vi "SDCP SMF Receiver and Transmitter - Live Plot - Obtain Data Points.vi"(4 "error in (no error)":errorcluster, 5 "Plot file path":path, 6 "Command":enum16{"Initialize", "Acquire", "Save"}(ring), 7 "Raw frame":T1) -> (0 "error out":errorcluster)   [LabVIEW 2020]
uses:
  <vilib>/Utility/file.llb/Write Delimited Spreadsheet (string).vi
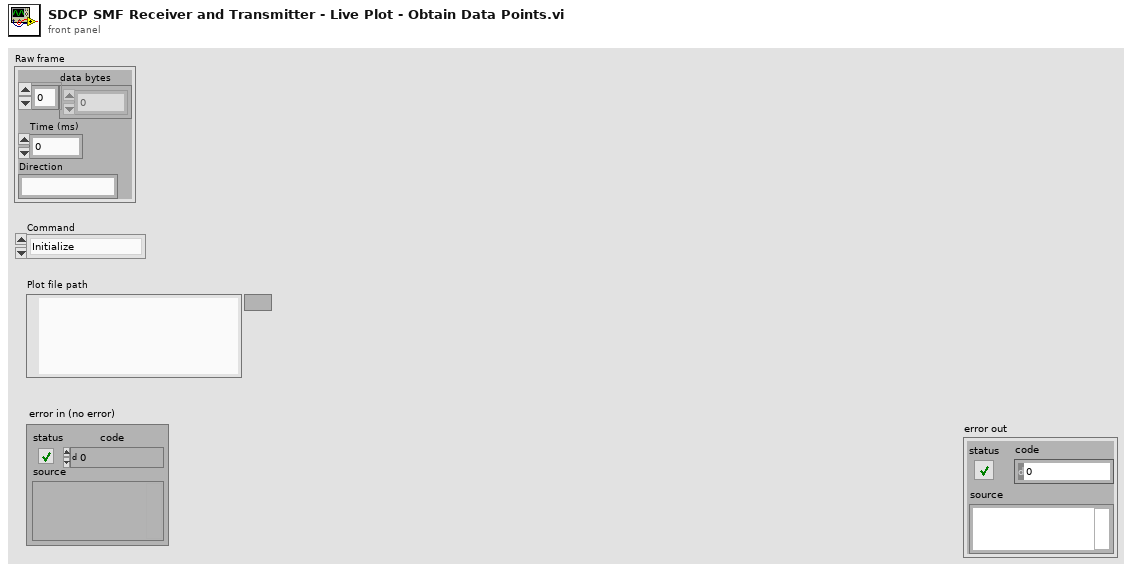
[diagram p1: front panel]
types:
  T1 = cluster{"data bytes":u8[], "Time (ms)":u32, "Direction":string}
  T2 = cluster{"Plot data":cluster{"X":dbl, "Y":dbl}[], "Plot name":string}
  T3 = cluster{"Plot data":cluster{"X":dbl, "Y":dbl}[], "Plot name":string}[]
  T4 = enum16{"open", "replace", "create", "open or create", "replace or create", "replace or create with confirmation"}
  T5 = typedef "SDCP - SMF parameter descriptors.ctl" = cluster{"Frame name":string, "Frame ID":i32, "Data type":string, "Start Position":i32, "Length":i32, "Factor":dbl, "Offset":dbl, "Parameter name":string, "Value":string}
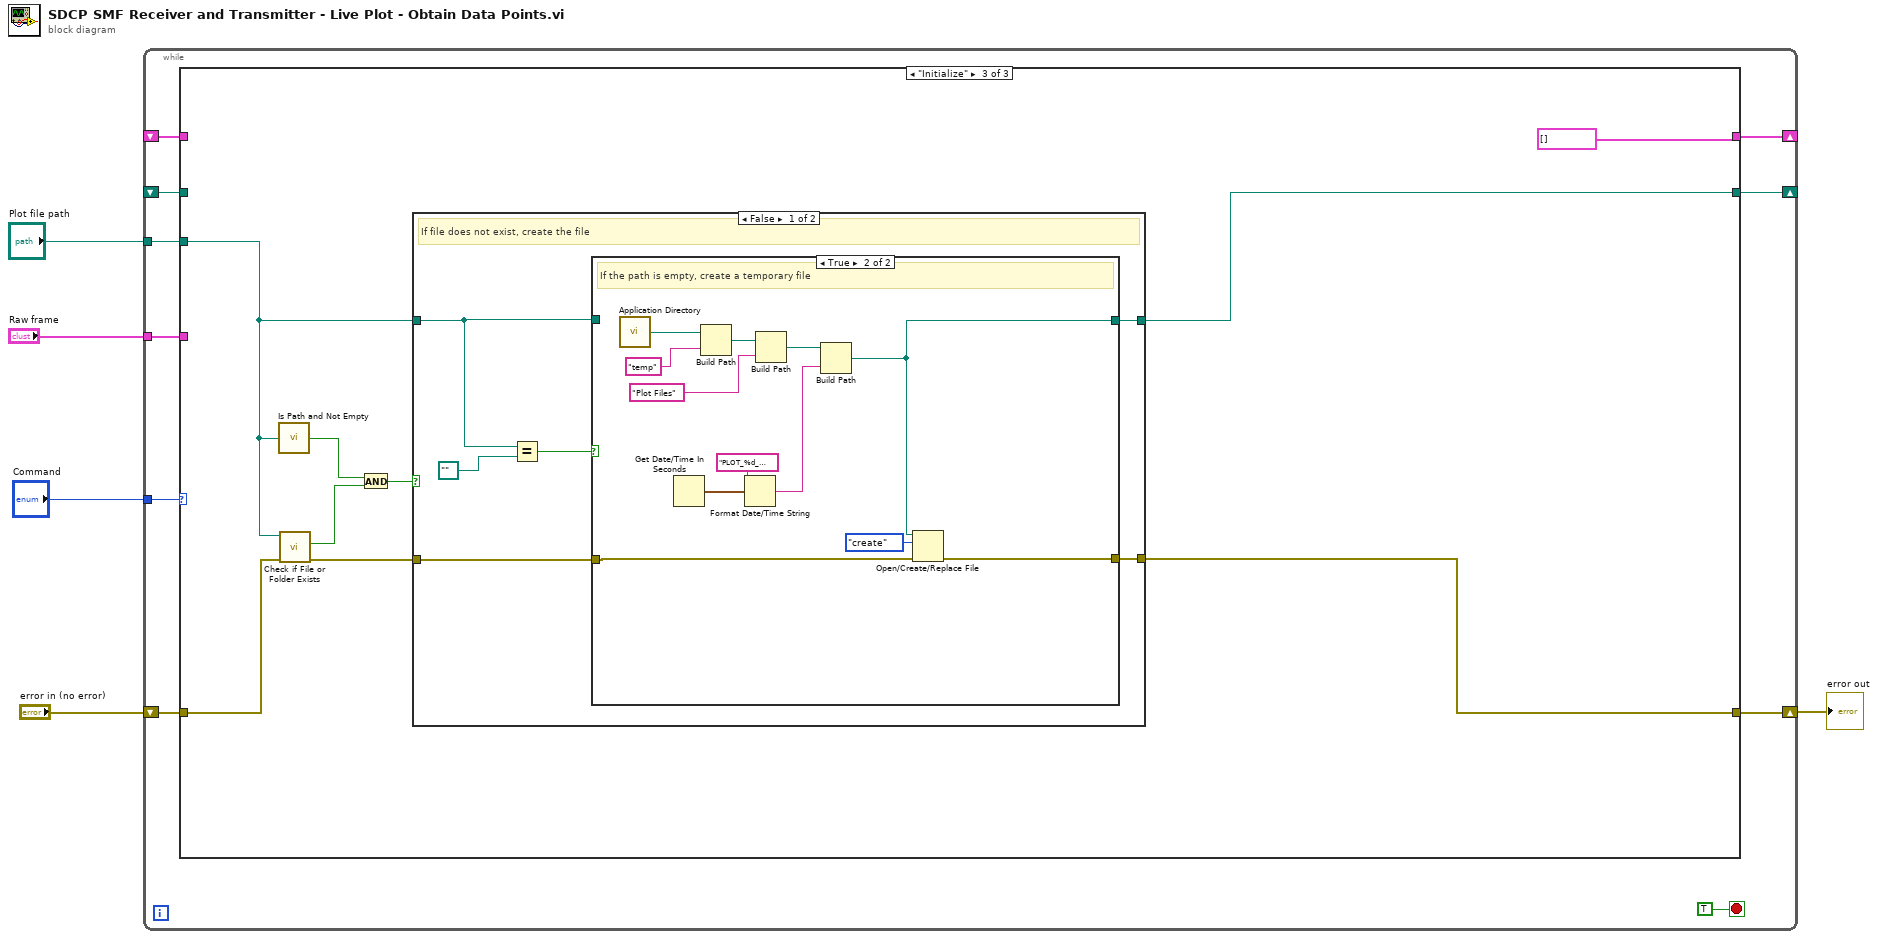
[diagram p0: block diagram]
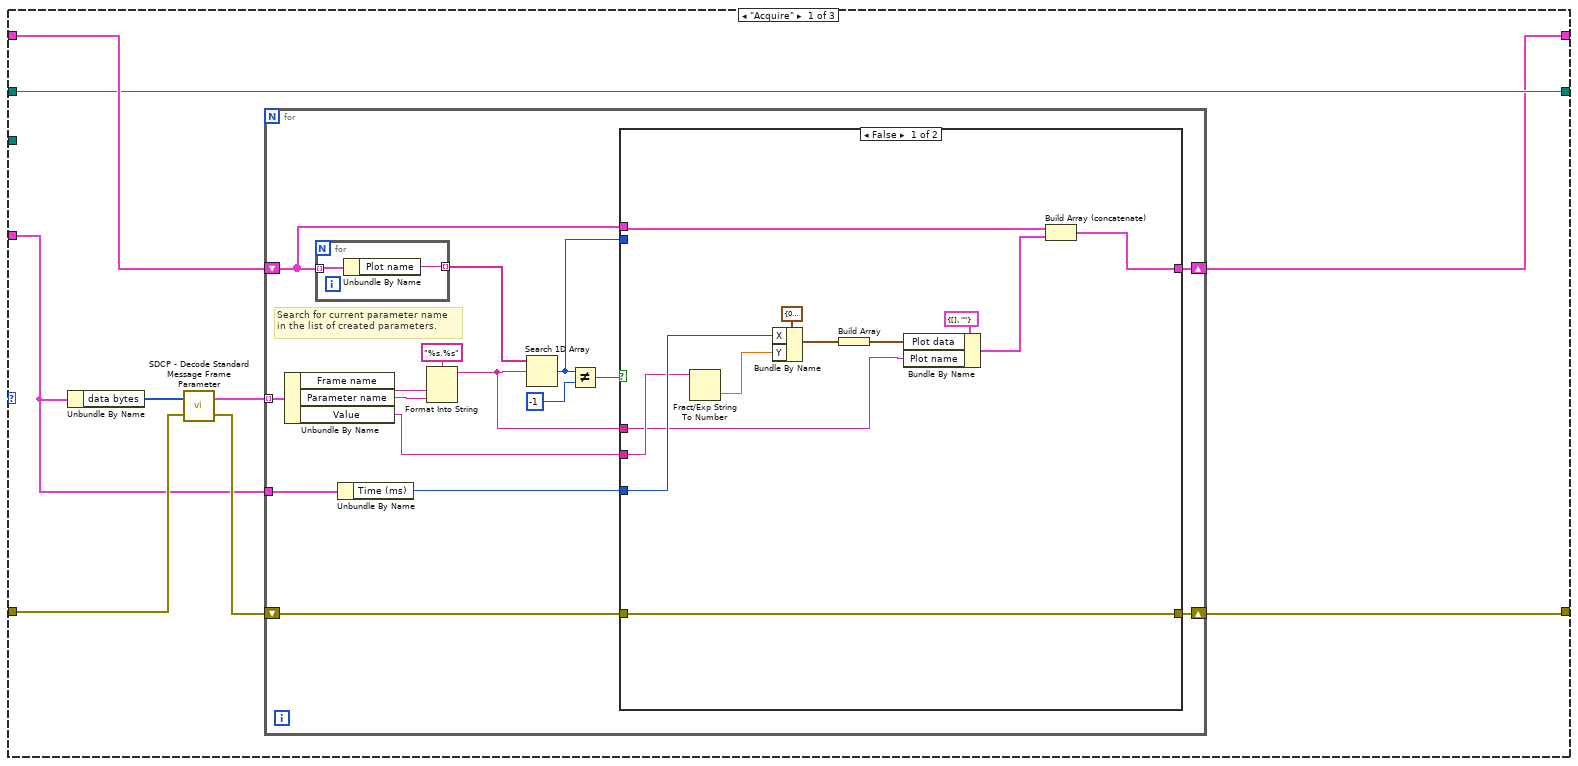
[diagram p2: hidden frame]
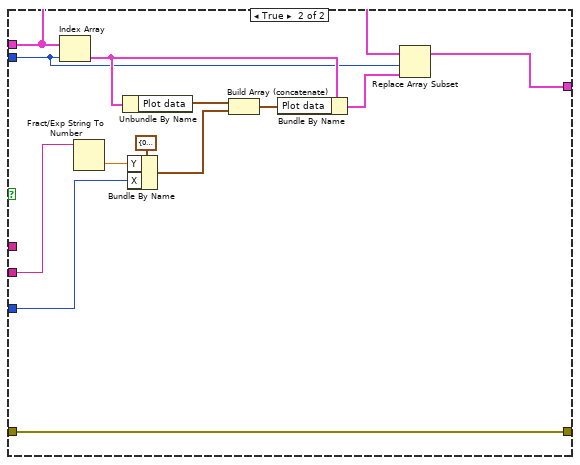
[diagram p3: hidden frame]
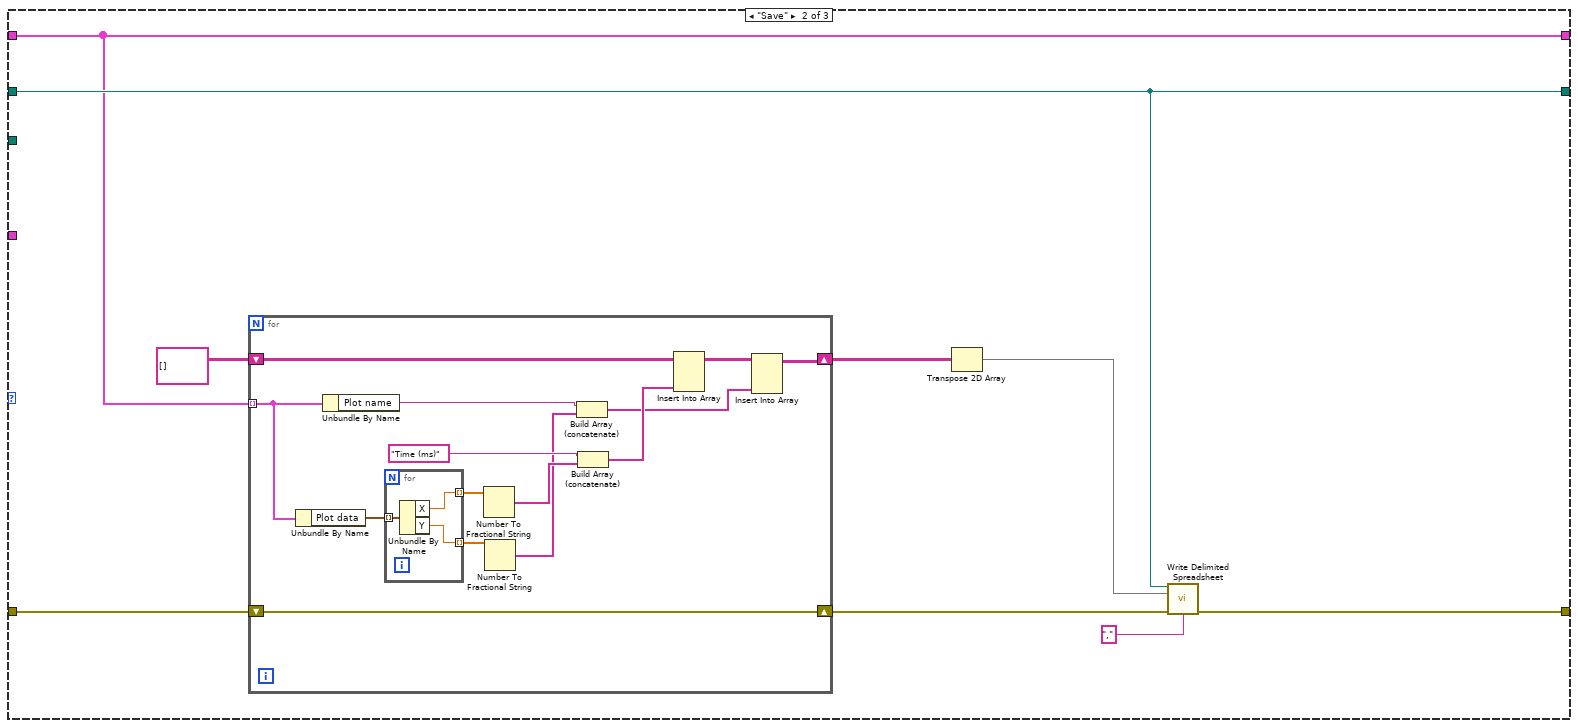
[diagram p4: hidden frame]
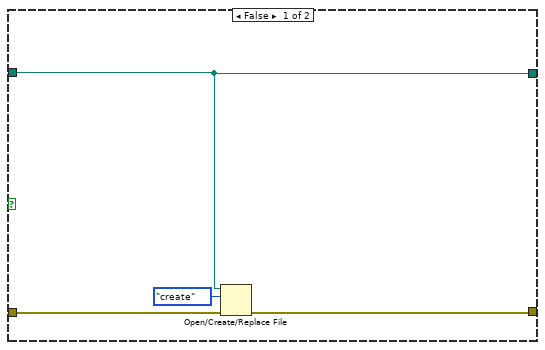
[diagram p5: hidden frame]
diagram:
  n1 = while {
    tunnel: "Raw frame" -> [w12]
    shift-right: [w13] -> w3
    shift-left: "error in (no error)" -> [w14]
    tunnel: "Command" -> [w11]
    shift-right: [w10] -> _
    shift-left: _ -> [w8]
    tunnel: "Plot file path" -> [w9]
    shift-right: [w7] -> _
    shift-left: _ -> [w6]
    stop <- TRUE stop-if-true
    n2 = case shown="\"Initialize\"" w11 {
      tunnel: w14 -> [w24 w74 w102]
      tunnel: [w19 w75 w95] -> w13
      tunnel: w12 -> [w20 _ _]
      tunnel: [w16 w68 T3 []] -> w10
      tunnel: w9 -> [_ _ w97]
      tunnel: w8 -> [w18 w68 _]
      tunnel: [w17 w69 w94] -> w7
      tunnel: w6 -> [w17 w69 _]
      frame "Acquire" {
        n3 = Unbundle By Name(w20) -> ("data bytes"=w23:u8[])
        n4 = call "SDCP - Decode Standard Message Frame Parameter.vi"("error in (no error)"=w24, "Bytes in"=w23) -> ("error out"=w22:errorcluster, "SMF Parameters out"=w21:T5[])
        n5 = for {
          shift-right: [w26] -> w19
          shift-left: w22 -> [w27]
          tunnel: w21 -> [w40] mode=indexing
          shift-right: [w28] -> w16
          shift-left: w18 -> [w33]
          tunnel: w20 -> [w30]
          # "Search for current parameter name\nin the list of created parameters."
          n6 = Unbundle By Name(w40) -> ("Frame name"=w38:string, "Parameter name"=w37:string, "Value"=w31:string)
          n7 = for {
            tunnel: w33 -> [w67] mode=indexing
            tunnel: [w66] -> w36 mode=indexing
            n8 = Unbundle By Name(w67) -> ("Plot name"=w66:string)
          }
          n9 = Unbundle By Name(w30) -> ("Time (ms)"=w29:u32)
          n10 = Format Into String(format string="%s.%s", w38, w37) -> (resulting string=w25:string)  [unwired: 2 in, 1 out]
          n11 = Search 1D Array(1D array=w36, element=w25) -> (index of element=w32:i32)  [unwired: 1 in]
          n12 = Not Equal?(x=w32, y=-1) -> (x != y?=w34:bool)
          n13 = case shown="False" w34 {
            tunnel: w33 -> [w52 w56]
            tunnel: w32 -> [_ w57]
            tunnel: w31 -> [w49 w62]
            tunnel: w29 -> [w50 w61]
            tunnel: [w42 w54] -> w28
            tunnel: w27 -> [w41 w53]
            tunnel: [w41 w53] -> w26
            tunnel: w25 -> [w44 _]
            frame False {
              n14 = Fract/Exp String To Number(string=w49) -> (number=w48:dbl)  [unwired: 3 in, 1 out]
              n15 = Bundle By Name(cluster=cluster{"X":dbl, "Y":dbl} {"X"=0.0, "Y"=0.0}, "X"=w50, "Y"=w48) -> (w46:cluster{"X":dbl, "Y":dbl})
              n16 = Build Array(w46) -> (w45:cluster{"X":dbl, "Y":dbl}[])
              n17 = Bundle By Name(cluster=T2 {"Plot data"=[], "Plot name"=""}, "Plot data"=w45, "Plot name"=w44) -> (w43:T2)
              n18 = Build Array (concatenate)(w52, w43) -> (w42:T3)
            }
            frame True {
              n19 = Index Array(array=w56, index=w57) -> (element=w59:T2)
              n20 = Fract/Exp String To Number(string=w62) -> (number=w63:dbl)  [unwired: 3 in, 1 out]
              n21 = Unbundle By Name(w59) -> ("Plot data"=w65:cluster{"X":dbl, "Y":dbl}[])
              n22 = Bundle By Name(cluster=cluster{"X":dbl, "Y":dbl} {"X"=0.0, "Y"=0.0}, "Y"=w63, "X"=w61) -> (w60:cluster{"X":dbl, "Y":dbl})
              n23 = Build Array (concatenate)(w65, w60) -> (w58:cluster{"X":dbl, "Y":dbl}[])
              n24 = Bundle By Name(cluster=w59, "Plot data"=w58) -> (w55:T2)
              n25 = Replace Array Subset(array=w56, new element=w55, index=w57) -> (w54:T3)
            }
          }
        }
      }
      frame "Save" {
        n26 = for {
          shift-right: [w82] -> w72
          shift-left: string[][] [] -> [w86]
          shift-right: [w81] -> w73
          shift-left: w74 -> [w81]
          tunnel: w68 -> [w77] mode=indexing
          n27 = Unbundle By Name(w77) -> ("Plot data"=w90:cluster{"X":dbl, "Y":dbl}[])
          n28 = Unbundle By Name(w77) -> ("Plot name"=w80:string)
          n29 = for {
            tunnel: w90 -> [w91] mode=indexing
            tunnel: [w93] -> w79 mode=indexing
            tunnel: [w92] -> w78 mode=indexing
            n30 = Unbundle By Name(w91) -> ("X"=w93:dbl, "Y"=w92:dbl)
          }
          n31 = Number To Fractional String(number=w79) -> (F-format string=w89:string[])  [unwired: 3 in]
          n32 = Number To Fractional String(number=w78) -> (F-format string=w87:string[])  [unwired: 3 in]
          n33 = Build Array (concatenate)(w80, w87) -> (w83:string[])
          n34 = Build Array (concatenate)("Time (ms)" ("element"), w89) -> (w85:string[])
          n35 = Insert Into Array(array=w86, new element=w85) -> (w84:string[][])  [unwired: 2 in]
          n36 = Insert Into Array(array=w84, new element=w83) -> (w82:string[][])  [unwired: 2 in]
        }
        n37 = Transpose 2D Array(2D array=w72) -> (transposed array=w70:string[][])
        n38 = call-poly <vilib>:"Write Delimited Spreadsheet.vi"("file path (dialog if empty)"=w69, "2D data"=w70, "error in (no error)"=w73, "delimiter (\\t)"="," ("delimiter (\\t)")) -> ("error out"=w75:errorcluster)  [unwired: 10 in, 1 out]
      }
      frame "Initialize" {
        n39 = call <vilib>:"Is Path and Not Empty.vi"("path"=w97) -> ("Is Path and Not Empty?"=w99:bool)  [unwired: 4 in]
        n40 = call <vilib>:"Check if File or Folder Exists.vi"("error in (no error)"=w102, "path"=w97) -> ("error out"=w101:errorcluster, "file or folder exists?"=w98:bool)  [unwired: 7 in, 1 out]
        n41 = And(x=w99, y=w98) -> (x .and. y?=w100:bool)
        n42 = case shown="False" w100 {
          tunnel: w101 -> [w107 w125]
          tunnel: w97 -> [w104 w126]
          tunnel: [w106 w126] -> w94
          tunnel: [w105 w125] -> w95
          frame False {
            # "If file does not exist, create the file"
            n43 = Equal?(x=w104, y=path "") -> (x = y?=w103:bool)
            n44 = case shown="True" w103 {
              tunnel: w107 -> [w111 w116]
              tunnel: [w109 w114] -> w106
              tunnel: [w110 w113] -> w105
              tunnel: w104 -> [w109 _]
              frame False {
                n45 = Open/Create/Replace File(file path (use dialog)=w109, error in=w111, operation (0:open)=T4."create") -> (error out=w110:errorcluster)  [unwired: 3 in, 2 out]
              }
              frame True {
                # "If the path is empty, create a temporary file"
                n46 = call <vilib>:"Application Directory.vi"() -> ("Application Directory"=w124:path)
                n47 = Get Date/Time In Seconds() -> (seconds since 1Jan1904=w120:timestamp)
                n48 = Build Path(base path=w124, name or relative path="temp") -> (appended path=w122:path)
                n49 = Format Date/Time String(time format string (%c)="PLOT_%d_%m_%Y__%H_%M_%S.csv", seconds (now)=w120) -> (date/time string=w117:string)  [unwired: 1 in]
                n50 = Build Path(base path=w122, name or relative path="Plot Files") -> (appended path=w118:path)
                n51 = Build Path(base path=w118, name or relative path=w117) -> (appended path=w114:path)
                n52 = Open/Create/Replace File(file path (use dialog)=w114, error in=w116, operation (0:open)=T4."create") -> (error out=w113:errorcluster)  [unwired: 3 in, 2 out]
              }
            }
          }
          frame True {
            # "If file exists, do nothing."
          }
        }
      }
    }
  }
  "error out" <- w3
